vi "WPI_InterruptWait.vi"(8 "error in (no error)":errorcluster, 9 "Ignore Previous Interrupts":bool, 10 "Timeout (ms)":i32=-1, 11 "InterruptRef":T1={"DevStatus"={"status"=FALSE, "code"=0, "source"=""}, "InterruptIndex"=enum."Invalid"}) -> (0 "error out":errorcluster, 1 "TimeStamp":dbl, 2 "Timed Out":bool, 3 "InterruptRef":T1={"DevStatus"={"status"=FALSE, "code"=0, "source"=""}, "InterruptIndex"=enum."Invalid"}, 4 "Falling Edge Interrupt":bool)   [LabVIEW 2017]
doc: "Specifies that the roboRIO waits for an interrupt. If the roboRIO receives an interrupt during the time you specify, this VI returns a <B>Timed Out</B> value of FALSE. You then can handle the interrupt as appropriate. If the roboRIO times out before receiving an interrupt, this VI returns a <B>Timed Out</B> value of TRUE. You can set this VI to wait for an interrupt indefinitely by setting <B>Timeout (ms)</B> to <B>-1</B>.\n\nThis software is licensed. Open the labview\\readme\\WPI Robotics Library Open Source License.txt file for more information."
uses:
  <vilib>/Rock Robotics/WPI/Interrupt/WPI_InterruptRef.ctl
  <vilib>/Rock Robotics/SystemInterfaces/Interrupt/FPGA_InterruptIndex.ctl
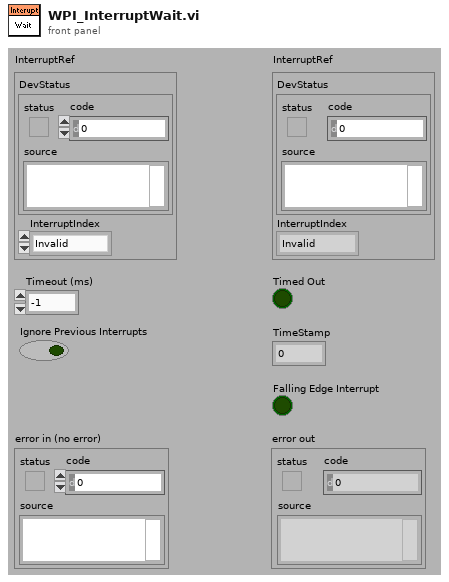
[diagram p1: front panel]
types:
  T1 = typedef "WPI_InterruptRef.ctl" = cluster{"DevStatus":errorcluster, "InterruptIndex":T2}
  T2 = typedef "FPGA_InterruptIndex.ctl" = enum8{"0", "1", "2", "3", "4", "5", "6", "7", "Invalid"}
  T3 = typedef "FPGA_InterruptRef.ctl" = cluster{"DevStatus":errorcluster, "Interrupt Index":T2}
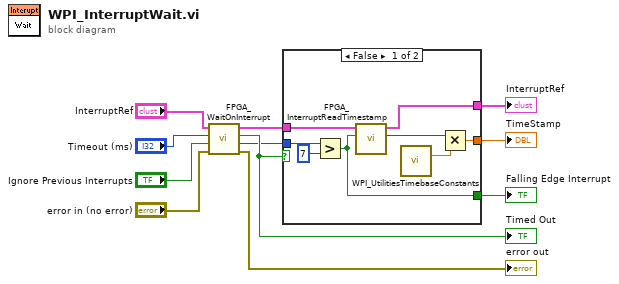
[diagram p0: block diagram]
diagram:
  n1 = call <vilib>:"FPGA_WaitOnInterrupt.vi"("error in (no error)"="error in (no error)", "Ignore Previous Interrupts"="Ignore Previous Interrupts", "Timeout (ms)"="Timeout (ms)", "InteruptRef"="InterruptRef") -> ("error out"=→"error out":errorcluster, "IRQ Asserted"=w2:i32, "Timed Out"=w4:bool, "InteruptRef"=w7:T3)  [unwired: 4 out]
  "Timed Out" <- w4
  n2 = case shown="False" w4 {
    tunnel: w7 -> [w19 w20]
    tunnel: [w17 _] -> w6
    tunnel: [w16 w20] -> w5
    tunnel: w2 -> [w14 _]
    tunnel: [w12 _] -> w1
    frame False {
      n3 = Greater?(x=w14, y=7) -> (0:w12:bool)
      n4 = call <vilib>:"FPGA_InterruptReadTimestamp.vi"("Falling Interrupt"=w12, "InteruptRef in"=w19) -> ("TimeStamp"=w18:u32, "InteruptRef out"=w16:T3)  [unwired: 1 in, 7 out]
      n5 = call <vilib>:"WPI_UtilitiesTimebaseConstants.vi"() -> ("1 MHz PWM clock"=w15:dbl)  [unwired: 13 in, 2 out]
      n6 = Multiply(x=w18, y=w15) -> (x*y=w17:dbl)
    }
    frame True {
    }
  }
  "InterruptRef" <- w5
  "TimeStamp" <- w6
  "Falling Edge Interrupt" <- w1
